vi "rect_scanning_cluster_fixed.vi"(9 "Slow Axis":i32, 10 "Fast Axis":i32, 11 "Scanning":T1={"Fast Axis Offset"=0.0, "Slow Axis Offset"=0.0, "Slow Axis Amp"=2.0, "Fast Axis Amp"=2.0, "Scan Pattern"=enum."Raster"} {"Fast Axis Amp" max=20 format="%#.2f"; "Slow Axis Amp" max=20 format="%#.2f"; "Slow Axis Offset" max=10 format="%#.2f"; "Fast Axis Offset" max=10 format="%#.2f"}) -> (3 "Scan Pattern 7":dbl[][](graph))   [LabVIEW 2014]
uses:
  Classes/Galvo/Scanning Cluster.ctl
  <vilib>/Analysis/NI_AALBase.lvlib
  Classes/Galvo/Galvo.lvclass
panel:
  out "Scan Pattern":cluster{dbl[], dbl[]}(graph)
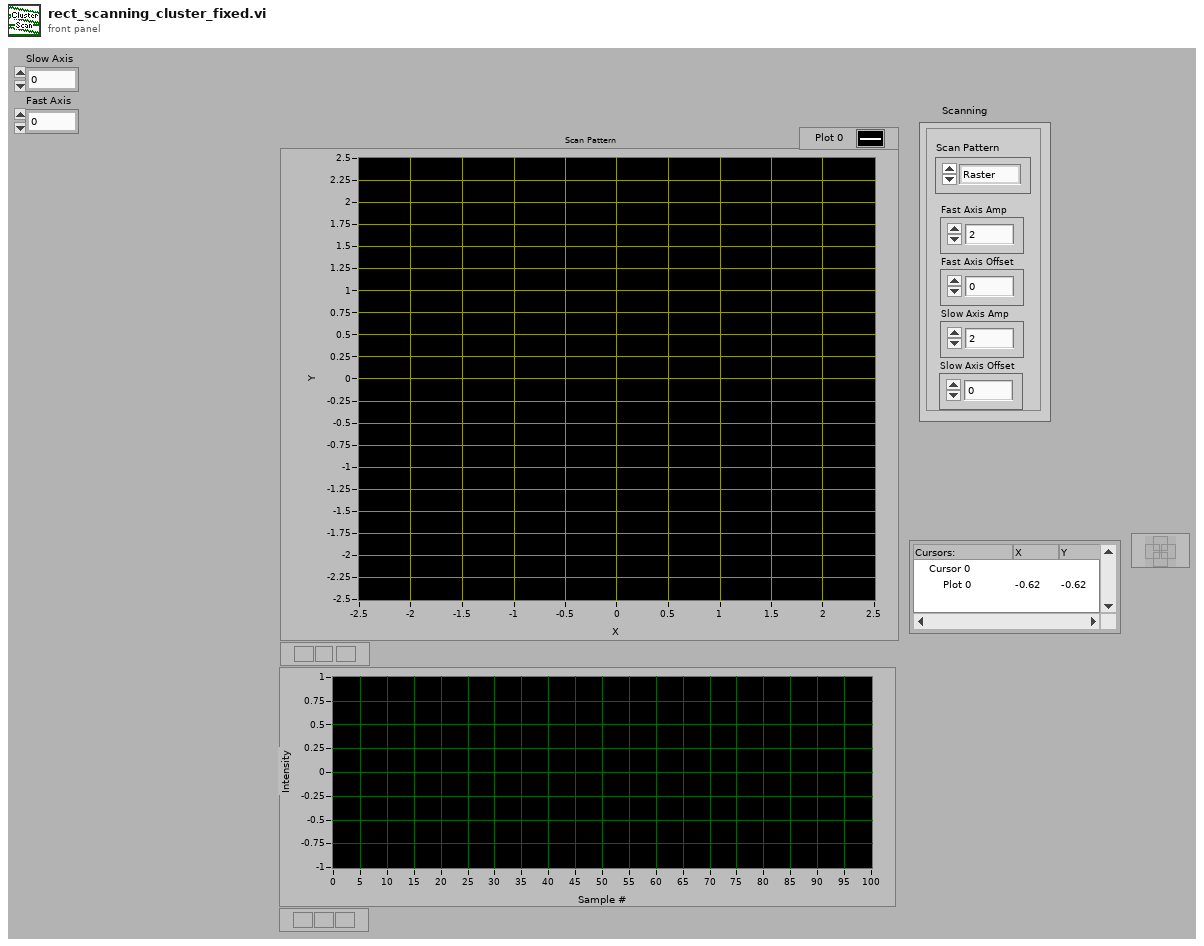
[diagram p1: front panel]
types:
  T1 = typedef "Galvo.lvclass/Scanning Cluster.ctl" = cluster{"Fast Axis Offset":sgl, "Slow Axis Offset":sgl, "Slow Axis Amp":sgl, "Fast Axis Amp":sgl, "Scan Pattern":enum16{"Raster"}}
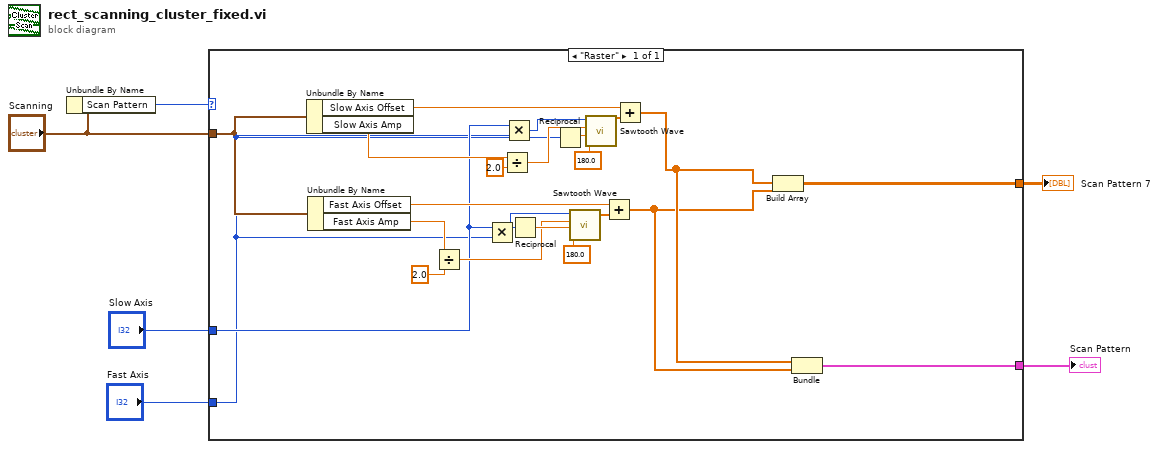
[diagram p0: block diagram]
diagram:
  n1 = Unbundle By Name("Scanning") -> ("Scan Pattern"=w3:enum16{"Raster"})
  n2 = case shown="\"Raster\"" w3 {
    tunnel: "Scanning" -> [w14]
    tunnel: [w10] -> w6
    tunnel: [w9] -> w5
    tunnel: "Slow Axis" -> [w8]
    tunnel: "Fast Axis" -> [w7]
    frame "Raster" {
      n3 = Unbundle By Name(w14) -> ("Slow Axis Offset"=w19:sgl, "Slow Axis Amp"=w22:sgl)
      n4 = Unbundle By Name(w14) -> ("Fast Axis Offset"=w29:sgl, "Fast Axis Amp"=w18:sgl)
      n5 = Divide(x=w18, y=2.0) -> (x/y=w12:dbl)
      n6 = Multiply(x=w8, y=w7) -> (x*y=w20:i32)
      n7 = Divide(x=w22, y=2.0 ("x")) -> (x/y=w13:dbl)
      n8 = Multiply(x=w8, y=w7) -> (x*y=w21:i32)
      n9 = Reciprocal(x=w20) -> (1/x=w25:dbl)
      n10 = Reciprocal(x=w7) -> (1/x=w24:dbl)
      n11 = call <vilib>:"Sawtooth Wave.vi"("samples"=w20, "amplitude"=w12, "frequency"=w25, "phase in"=180.0 ("S_phase")) -> ("sawtooth wave"=w27:dbl[])  [unwired: 1 in, 2 out]
      n12 = call <vilib>:"Sawtooth Wave.vi"("samples"=w21, "amplitude"=w13, "frequency"=w24, "phase in"=180.0) -> ("sawtooth wave"=w28:dbl[])  [unwired: 1 in, 2 out]
      n13 = Add(x=w29, y=w27) -> (x+y=w16:dbl[])
      n14 = Add(x=w19, y=w28) -> (x+y=w17:dbl[])
      n15 = Build Array(w17, w16) -> (w9:dbl[][])
      n16 = Bundle(w17, w16) -> (w10:cluster{dbl[], dbl[]})  [unwired: 1 out]
    }
  }
  "Scan Pattern 7" <- w5
  "Scan Pattern" <- w6
